vi "AutoFeedForwardConversion.vi"(1 "Target Velocity (in/s)":dbl) -> (0 "Equivalent Joystick Command (ul)":dbl)   [LabVIEW 2019]
doc: "Converts the feed-forward path goal velocity from inches/sec to a unitless drive command. This VI is intended for use with the FRC 4265 Autonomous Path Planner and the pure-pursuit algorithm. The input is in inches per second and the output is a unitless equivalent joystick command."
uses:
  constants.vi
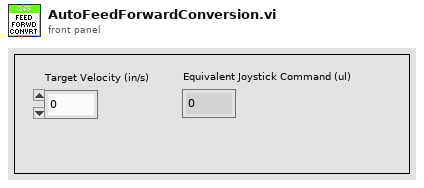
[diagram p1: front panel]
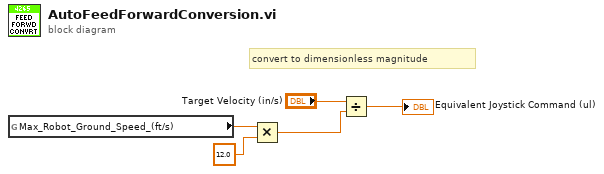
[diagram p0: block diagram]
diagram:
  # "convert to dimensionless magnitude"
  n1 = global read "constants.vi" "Max_Robot_Ground_Speed_(ft/s)"() -> (w1:dbl)
  n2 = Multiply(x=w1, y=12.0) -> (x*y=w2:dbl)
  n3 = Divide(x="Target Velocity (in/s)", y=w2) -> (x/y=→"Equivalent Joystick Command (ul)":dbl)
